vi "Update Energy Storage Parameter.vi"(10 "Energy Storage Parameters":T1, 11 "Optimization in":refnum<class "Optimization.lvclass">) -> (3 "Optimization out":refnum<class "Optimization.lvclass">)   [LabVIEW 2016, in "Optimization Framework.lvlib" / "Optimization.lvclass"]
uses:
  Optimization.lvclass
  Controls/Optimization Parameters Energy Storage.ctl
  Controls/Device Control Capabilities.ctl
  Optimization.lvclass/Optimization.ctl
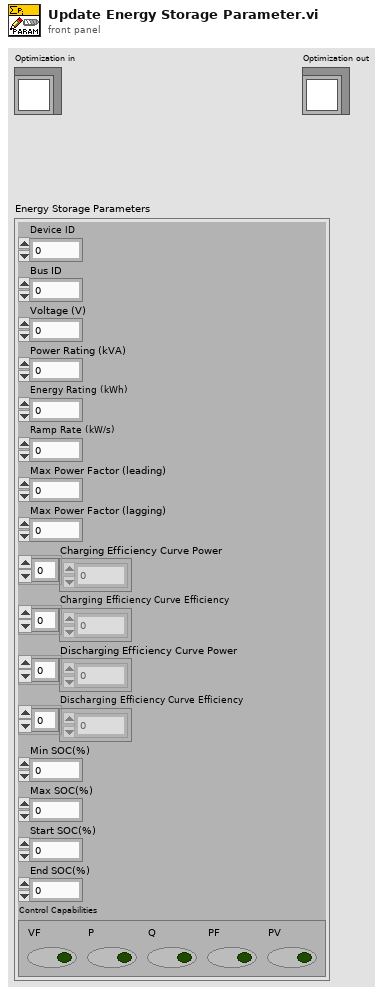
[diagram p1: front panel]
types:
  T1 = typedef "Optimization Framework.lvlib/Optimization.lvclass/Optimization Parameters Energy Storage.ctl" = cluster{"Device ID":u64, "Bus ID":u16, "Voltage (V)":dbl, "Power Rating (kVA)":dbl, "Energy Rating (kWh)":dbl, "Ramp Rate (kW/s)":dbl, "Max Power Factor (leading)":dbl, "Max Power Factor (lagging)":dbl, "Charging Efficiency Curve Power":dbl[], "Charging Efficiency Curve Efficiency":dbl[], "Discharging Efficiency Curve Power":dbl[], "Discharging Efficiency Curve Efficiency":dbl[], "Min SOC(%)":dbl, "Max SOC(%)":dbl, "Start SOC(%)":dbl, "End SOC(%)":dbl, "Control Capabilities":T2}
  T2 = typedef "Optimization Framework.lvlib/Optimization.lvclass/Device Control Capabilities.ctl" = cluster{"VF":bool, "P":bool, "Q":bool, "PF":bool, "PV":bool}
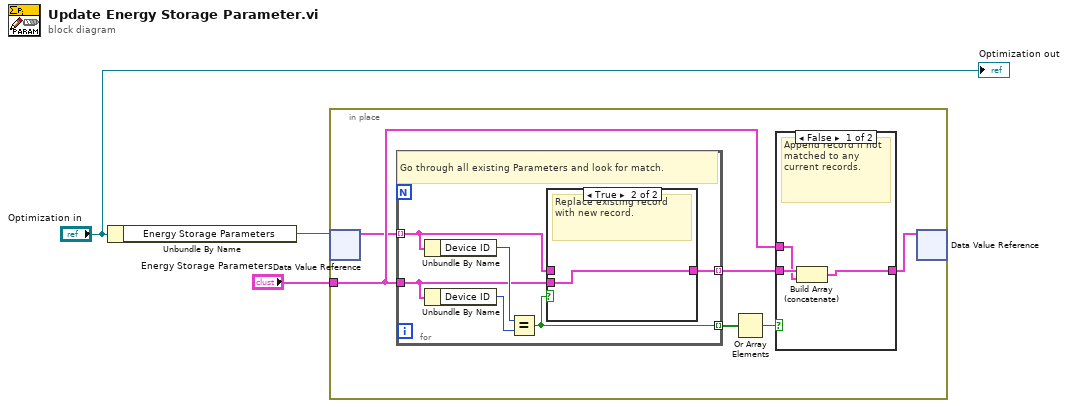
[diagram p0: block diagram]
diagram:
  n1 = Unbundle By Name("Optimization in") -> ("Energy Storage Parameters"=w2:refnum<data-value>)
  n2 = in-place {
    in-place-border: "Energy Storage Parameters" -> [w6]
    n3 = in-place-dvr #1(w2) -> (w5:T1[])  [unwired: 1 out]
    n4 = for {
      tunnel: w5 -> [w15] mode=indexing
      tunnel: w6 -> [w16]
      tunnel: [w17] -> w9 mode=indexing
      tunnel: [w14] -> w7 mode=indexing
      # "Go through all existing Parameters and look for match."
      n5 = Unbundle By Name(w15) -> ("Device ID"=w19:u64)
      n6 = Unbundle By Name(w16) -> ("Device ID"=w18:u64)
      n7 = Equal?(x=w19, y=w18) -> (x = y?=w14:bool)
      n8 = case shown="True" w14 {
        tunnel: [w20 w21] -> w17
        tunnel: w16 -> [_ w21]
        tunnel: w15 -> [w20 _]
        frame False {
          # "Keep existing record."
        }
        frame True {
          # "Replace existing record with new record."
        }
      }
    }
    n9 = Or Array Elements(Boolean array=w7) -> (logical OR=w8:bool)
    n10 = case shown="False" w8 {
      tunnel: w6 -> [w11 _]
      tunnel: w9 -> [w12 w13]
      tunnel: [w10 w13] -> w4
      frame False {
        # "Append record if not matched to any current records."
        n11 = Build Array (concatenate)(w12, w11) -> (w10:T1[])
      }
      frame True {
        # "Record was replaced, pass through."
      }
    }
    n12 = in-place-dvr #1(w4) -> ()  [unwired: 2 out]
  }
  "Optimization out" <- "Optimization in"
